vi "Go.vi"(9 "Timing Values":dbl[](array[numeric]), 10 "Control In":T1, 11 "CAD Dispense in":refnum<class "CAD Dispense.lvclass">) -> (2 "Control Out":T1, 3 "CAD Dispense Out":refnum<class "CAD Dispense.lvclass">)   [LabVIEW 2020, in "CAD Dispense.lvclass"]
uses:
  CAD Dispense.lvclass
  Controller/Motion/Motion.lvclass
  Controller/Dispenser/Dispenser.lvclass
  Aerotech.lvlib
  Program Files (x86)/Aerotech/A3200/LabVIEW/2010/Motion/MoveIncSingle.vi
  Controller/Controllers.ctl
  Controller/Controller.lvclass
  Controller/I-O/I-O.lvclass
  C:/Program Files (x86)/Aerotech/A3200/LabVIEW/2010/Bin/Aerotech.A3200.dll
  Program Files (x86)/Aerotech/A3200/LabVIEW/2010/Bin/Aerotech.A3200.dll
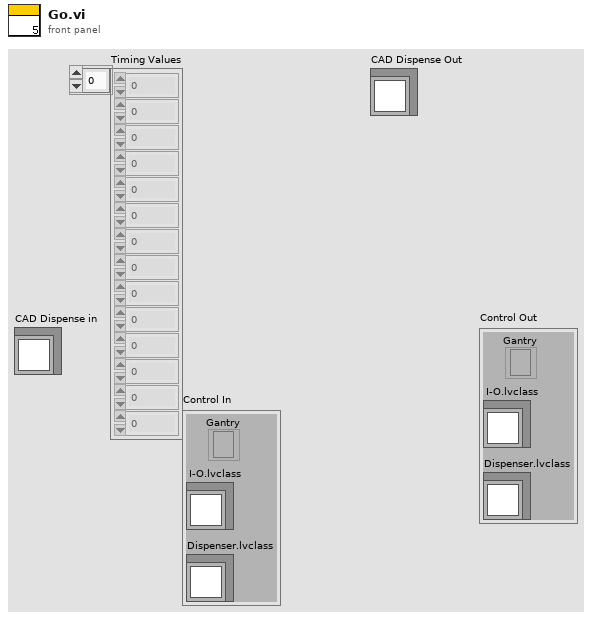
[diagram p1: front panel]
types:
  T1 = typedef "Controller.lvclass/Controllers.ctl" = cluster{"I-O.lvclass":refnum<class "I-O.lvclass">, "Dispenser.lvclass":refnum<class "Dispenser.lvclass">, "Gantry":refnum<k24>}
  T2 = cluster{"Motion":dbl[][], "Center":dbl[], "CW/CCW":dbl, "Dispense Type":enum16{"N-gon", "Square", "Arc", "Dot", "Line", "Circle"}}[]
  T3 = cluster{"Motion":dbl[][], "Center":dbl[], "CW/CCW":dbl, "Dispense Type":enum16{"N-gon", "Square", "Arc", "Dot", "Line", "Circle"}}
  T4 = typedef "ControllerDiagPacket.ctl" = cluster{"Number of Diag Packets":i32, "Axes":T5[], "error":errorcluster}
  T5 = typedef "AxisDiagPacket.ctl" = cluster{"Axis Name":string, "Analog Input 0":dbl, "Analog Input 1":dbl, "Axis Fault (num)":i32, "Axis Fault (str)":string, "Axis Fault (bits)":cluster{"AmplifierFault":bool, "AmplifierTemperatureFault":bool, "CcwEndOfTravelLimitFault":bool, "CcwSoftwareLimitFault":bool, "CommunicationLostFault":bool, "CwEndOfTravelLimitFault":bool, "CwSoftwareLimitFault":bool, "EmergencyStopFault":bool, "EncoderFault":bool, "ExternalFault":bool, "FeedbackScalingFault":bool, "GantryMisalignFault ":bool, "HallSensorFault":bool, "InPositionTimeoutFault":bool, "InternalFault":bool, "MarkerSearchFault":bool, "MaxVelocityCommandFault":bool, "MissedInterruptFault":bool, "MotorTemperatureFault":bool, "None":bool, "OverCurrentFault":bool, "PositionErrorFault":bool, "PositionFeedbackFault":bool, "PowerSupplyFault":bool, "ProbeInputFault":bool, "SafeZoneFault":bool, "VelocityErrorFault":bool, "VelocityFeedbackFault":bool, "VoltageClampFault":bool}, "Axis Status (num)":i32, "Axis Status (str)":string, "Axis Status (bits)":cluster{"BacklashActive":bool, "CalibrationEnabled1D":bool, "CalibrationEnabled2D":bool, "CommandValid":bool, "DriveAbortPending":bool, "DrivePending":bool, "Enabling":bool, "GainMappingEnabled":bool, "GantryAligned":bool, "GantryRealigning":bool, "Homed":bool, "Homing":bool, "IFOVEnabled":bool, "JogGenerating":bool, "Jogging":bool, "JoystickControl":bool, "MasterSlaveControl":bool, "MotionBlocked":bool, "MotionClamped":bool, "MoveDone":bool, "None":bool, "NotVirtual":bool, "Profiling":bool, "Stability0":bool, "Stability1":bool, "TrajectoryFiltering":bool, "WaitDone":bool}, "Current Command":sgl, "Current Error":sgl, "Current Feedback":sgl, "Digital Inputs":i32, "Digital Outputs":i32, "Drive Status":i32, "Drive Status (str)":string, "Drive Status (bits)":cluster{"AccelerationPhase":bool, "AutofocusActive":bool, "BrakeOutput":bool, "CcwEndOfTravelLimitInput":bool, "CosineEncoderError":bool, "CurrentClamp":bool, "CwEndOfTravelLimitInput":bool, "DecelerationPhase":bool, "DualLoopActive":bool, "EmergencyStopInput":bool, "Enabled":bool, "EncoderClipping":bool, "GalvoCalibrationEnabled":bool, "GalvoPowerCorrection":bool, "HallAInput":bool, "HallBInput":bool, "HallCInput":bool, "HighResolutionMode":bool, "HomeLimitInput":bool, "InPosition":bool, "InPosition2":bool, "MarkerInput":bool, "MarkerLatch":bool, "MoveActive":bool, "NoMotorSupply":bool, "None":bool, "PowerLimiting":bool, "ProgrammingFlash":bool, "ProgrammingMXH":bool, "PSOHaltLatch":bool, "ServoControl":bool, "SineEncoderError":bool}, "Position Feedback Auxiliary":dbl, "Position Command":dbl, "Position Error":dbl, "Position Feedback":dbl, "Program Position Command":dbl, "Program Position Error":dbl, "Program Position Feedback":dbl, "Velocity Command":dbl, "Velocity Error":dbl, "Velocity Feedback":dbl}
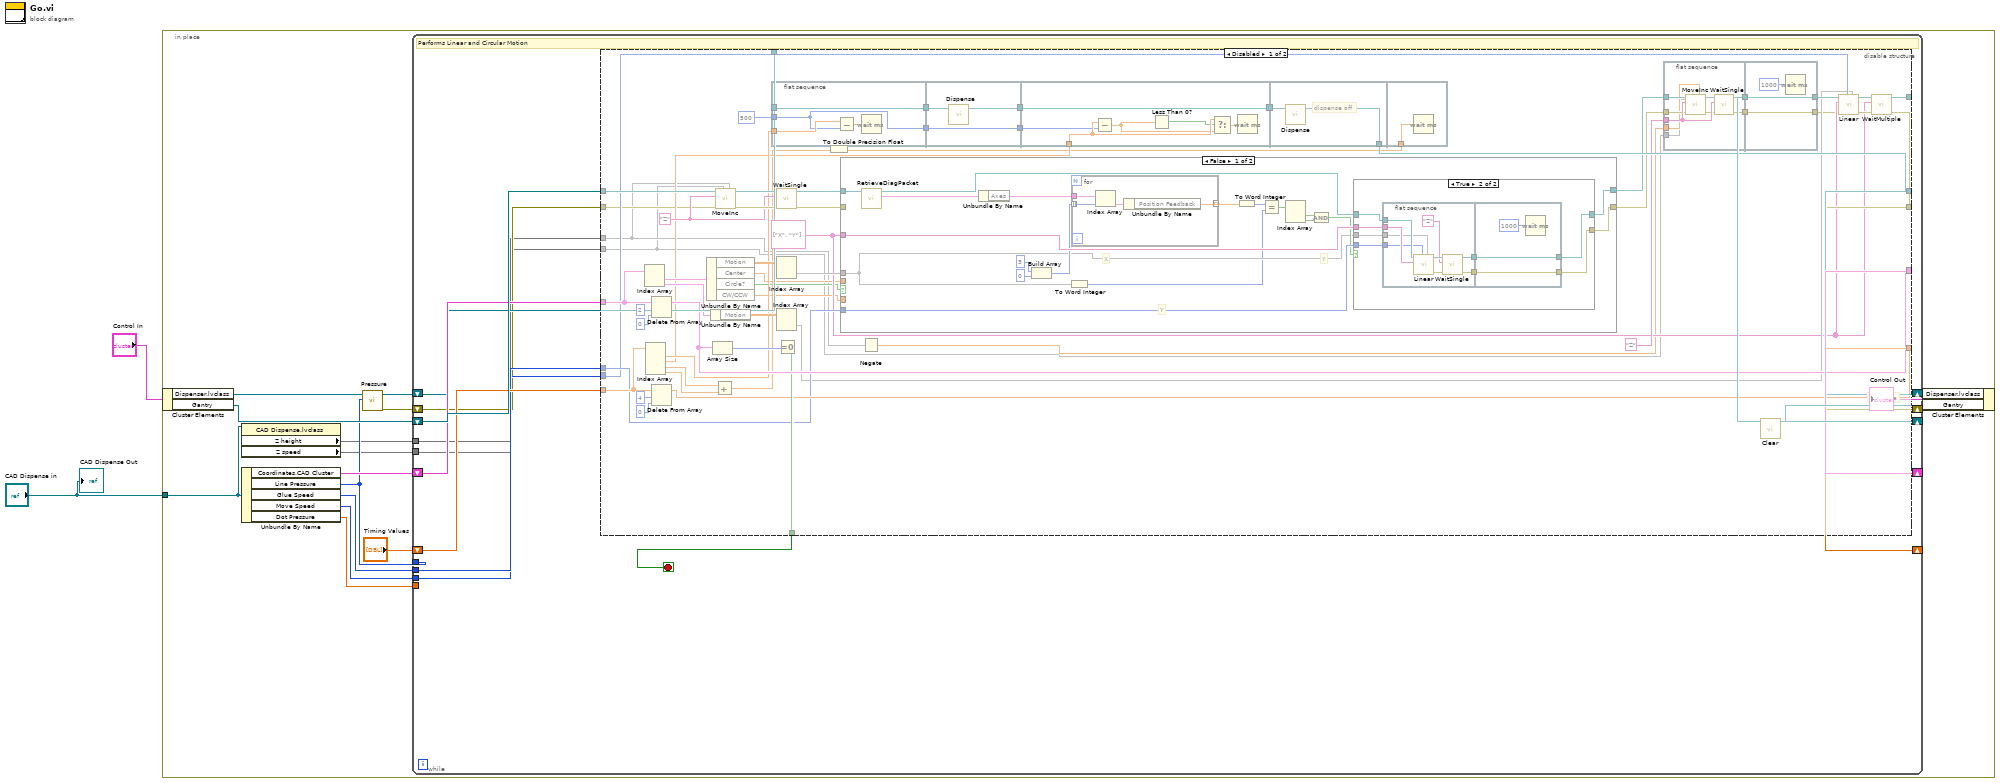
[diagram p0: block diagram]
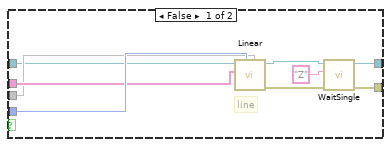
[diagram p2: hidden frame]
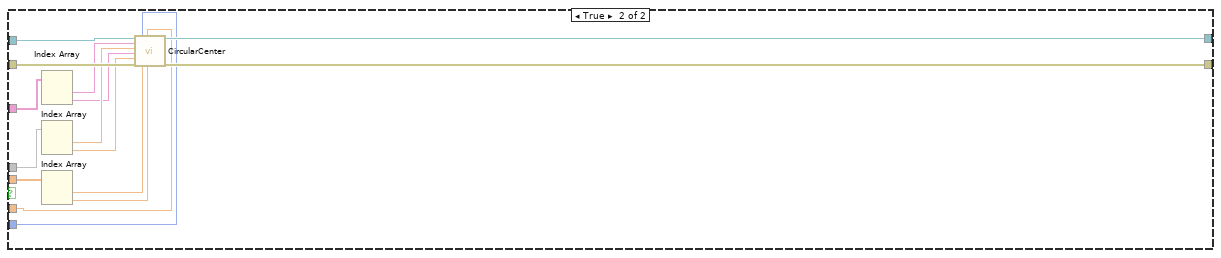
[diagram p3: hidden frame]
diagram:
  n1 = in-place {
    in-place-border: "CAD Dispense in" -> [w6]
    n2 = in-place-cluster #1("Control In") -> ("Dispenser.lvclass"=w18:refnum<class "Dispenser.lvclass">, "Gantry"=w15:refnum<k24>)
    n3 = property class="CAD Dispense.lvclass"(reference=w6) -> ("Z height"=w5, "Z speed"=w4)  [unwired: 1 in, 2 out]
    n4 = Unbundle By Name(w6) -> ("Coordinates.CAD Cluster"=w17:T2, "Line Pressure"=w7:i64, "Glue Speed"=w11:i32, "Move Speed"=w10:i32, "Dot Pressure"=w8:dbl)
    n5 = call-dynamic "Pressure.vi"("Pressure"=w7, "Dispenser in"=w18) -> ("error out"=w9:errorcluster, "Dispenser out"=w13:refnum<class "Dispenser.lvclass">)  [unwired: 8 in]
    n6 = while {
      shift-right: [w26] -> w19
      shift-left: w13 -> [w29]
      shift-right: [w30] -> w16
      shift-left: w15 -> [w34]
      shift-right: [w32] -> _
      shift-left: w17 -> [w33]
      shift-right: [w27] -> _
      shift-left: "Timing Values" -> [w28]
      tunnel: w11 -> [w25]
      tunnel: w10 -> [w24]
      shift-right: [w22] -> _
      shift-left: w9 -> [w23]
      tunnel: w8 -> [_]
      tunnel: w7 -> [_]
      tunnel: w5 -> [w21]
      tunnel: w4 -> [w20]
      stop <- w31 stop-if-true
      # "Performs Linear and Circular Motion"
      n7 = disable-structure shown="Disabled" {
        disable-tunnel: w34 -> [w83 _]
        disable-tunnel: w33 -> [w82 _]
        disable-tunnel: [w81 _] -> w32
        disable-tunnel: [w80 _] -> w31
        disable-tunnel: [w79 _] -> w30
        disable-tunnel: w29 -> [w78 _]
        disable-tunnel: w28 -> [w77 _]
        disable-tunnel: [w76 _] -> w27
        disable-tunnel: [w75 _] -> w26
        disable-tunnel: w25 -> [w74 _]
        disable-tunnel: w24 -> [w73 _]
        disable-tunnel: w23 -> [w42 _]
        disable-tunnel: [w41 _] -> w22
        disable-tunnel: w21 -> [w37 _]
        disable-tunnel: w20 -> [w35 _]
        frame Disabled {
          w55 = string[] ["X", "Y"] ("axis names")
          w61 = "Z" ("axis name")
          # "dispense"
          n8 = Index Array(array=w82) -> (element #1=w72:T3, element #2=w69:T3)  [unwired: 2 in]
          n9 = Index Array(array=w77) -> (element #1=w54:dbl, element #2=w53:dbl, element #3=w52:dbl, element #4=w51:dbl)  [unwired: 4 in]
          n10 = Delete From Array(array=w82, length=2, index=0) -> (array with subset deleted=w81:T2)  [unwired: 1 out]
          n11 = Delete From Array(array=w77, length=4, index=0) -> (array with subset deleted=w76:dbl[])  [unwired: 1 out]
          n12 = Unbundle By Name(w72) -> ("Motion"=w71:dbl[][], "Center"=w47:dbl[], "Circle?"=w46:bool, "CW/CCW"=w45:dbl)
          n13 = Unbundle By Name(w69) -> ("Motion"=w68:dbl[][])
          n14 = Array Size(array=w81) -> (size(s)=w64:i32)
          n15 = Add(x=w52, y=w51) -> (x+y=w50:dbl)
          n16 = call-poly "MoveInc.vi"("distance"=w37, "speed"=w35, "error in (no error)"=w42, "axis name"=w61, "controller in"=w83) -> ("error out"=w62:errorcluster, "controller out"=w63:refnum<k24>)  [unwired: 5 in]
          n17 = flat-sequence {
            tunnel: w54 -> [w171]
            tunnel: w78 -> [w173]
            tunnel: [w173] -> w90
            tunnel: 500 -> [w170]
            tunnel: [w170] -> w89
            tunnel: w90 -> [w176]
            tunnel: [w175] -> w88
            tunnel: w89 -> [w174]
            tunnel: [w174] -> w87
            tunnel: w53 -> [w182]
            tunnel: w88 -> [w177]
            tunnel: [w177] -> w86
            tunnel: w87 -> [w179]
            tunnel: w86 -> [w184]
            tunnel: [w183] -> w75
            tunnel: w50 -> [w185]
            frame #0 {
              n18 = Subtract(x=w171, y=w170) -> (x-y=w172:dbl)
              n19 = Wait (ms)(milliseconds to wait=w172) -> ()  [unwired: 1 out]
            }
            frame #1 {
              n20 = call-dynamic "Dispense.vi"("Dispenser in"=w176) -> ("Dispenser out"=w175:refnum<class "Dispenser.lvclass">)  [unwired: 9 in, 1 out]
            }
            frame #2 {
              n21 = Subtract(x=w182, y=w179) -> (x-y=w181:dbl)
              n22 = Less Than 0?(x=w181) -> (x < 0?=w178:bool)
              n23 = Select(t=w182, s=w178, f=w181) -> (s? t:f=w180:dbl)
              n24 = Wait (ms)(milliseconds to wait=w180) -> ()  [unwired: 1 out]
            }
            frame #3 {
              # "dispense off"
              n25 = call-dynamic "Dispense.vi"("Dispenser in"=w184) -> ("Dispenser out"=w183:refnum<class "Dispenser.lvclass">)  [unwired: 9 in, 1 out]
            }
            frame #4 {
              n26 = Wait (ms)(milliseconds to wait=w185) -> ()  [unwired: 1 out]
            }
          }
          n27 = call "WaitSingle.vi"("error in (no error)"=w62, "axis name"=w61, "controller in"=w63) -> ("error out"=w60:errorcluster, "controller out"=w38:refnum<k24>)  [unwired: 6 in, 1 out]
          n28 = Index Array(array=w71) -> (element=w70:dbl[])  [unwired: 2 in]
          n29 = Index Array(array=w68) -> (element=w67:dbl[])  [unwired: 2 in]
          n30 = Equal To 0?(x=w64) -> (x = 0?=w80:bool)
          n31 = To Double Precision Float() -> ()  [unwired: 1 in, 1 out]
          n32 = case shown="False" w46 {
            tunnel: w74 -> [w121 w165]
            tunnel: w70 -> [w106 w160]
            tunnel: w60 -> [_ w168]
            tunnel: [w118 w169] -> w40
            tunnel: [w120 w167] -> w39
            tunnel: w55 -> [w119 w166]
            tunnel: w47 -> [_ w163]
            tunnel: w45 -> [_ w164]
            tunnel: w38 -> [w107 w155]
            frame False {
              # "Y"
              # "X"
              # "Y"
              n33 = call "RetrieveDiagPacket.vi"("Controller In"=w107) -> ("ControllerDiagPacket"=w117:T4, "Controller Out"=w108:refnum<k24>)  [unwired: 8 in, 1 out]
              n34 = Unbundle By Name(w117) -> ("Axes"=w116:T5[])
              n35 = Build Array(3, 0) -> (w115:i32[])
              n36 = To Word Integer(number=w106) -> (16bit integer=w103:i16[])
              n37 = for {
                tunnel: w116 -> [w124]
                tunnel: [w125] -> w105 mode=indexing
                tunnel: w115 -> [w122] mode=indexing
                n38 = Index Array(array=w124, index=w122) -> (element=w123:T5)
                n39 = Unbundle By Name(w123) -> ("Position Feedback"=w125:dbl)
              }
              n40 = To Word Integer(number=w105) -> (16bit integer=w104:i16[])
              n41 = Equal?(x=w104, y=w103) -> (x = y?=w112:bool[])
              n42 = Index Array(array=w112) -> (element #1=w111:bool, element #2=w110:bool)  [unwired: 2 in]
              n43 = And(x=w111, y=w110) -> (x .and. y?=w109:bool)
              n44 = case shown="True" w109 {
                tunnel: w121 -> [w134 w139]
                tunnel: [w133 w135] -> w120
                tunnel: w119 -> [w132 w141]
                tunnel: [w131 w137] -> w118
                tunnel: w106 -> [w130 w140]
                tunnel: w108 -> [w126 w142]
                frame False {
                  # "line"
                  n45 = call "Linear.vi"("distances"=w130, "speed"=w134, "axis names"=w132, "controller in"=w126) -> ("error out"=w127:errorcluster, "controller out"=w129:refnum<k24>)  [unwired: 6 in]
                  n46 = call "WaitSingle.vi"("error in (no error)"=w127, "axis name"="Z", "controller in"=w129) -> ("error out"=w133:errorcluster, "controller out"=w131:refnum<k24>)  [unwired: 6 in, 1 out]
                }
                frame True {
                  n47 = flat-sequence {
                    tunnel: w142 -> [w148]
                    tunnel: w141 -> [w147]
                    tunnel: w140 -> [w146]
                    tunnel: w139 -> [w145]
                    tunnel: [w144] -> w138
                    tunnel: [w143] -> w136
                    tunnel: w138 -> [w153]
                    tunnel: [w153] -> w137
                    tunnel: w136 -> [w152]
                    tunnel: [w152] -> w135
                    frame #0 {
                      n48 = call "Linear.vi"("distances"=w146, "speed"=w145, "axis names"=w147, "controller in"=w148) -> ("error out"=w149:errorcluster, "controller out"=w151:refnum<k24>)  [unwired: 6 in]
                      n49 = call "WaitSingle.vi"("error in (no error)"=w149, "axis name"="Z", "controller in"=w151) -> ("error out"=w143:errorcluster, "controller out"=w144:refnum<k24>)  [unwired: 6 in, 1 out]
                    }
                    frame #1 {
                      n50 = Wait (ms)(milliseconds to wait=u32 1000) -> ()  [unwired: 1 out]
                    }
                  }
                }
              }
            }
            frame True {
              n51 = Index Array(array=w166) -> (element #1=w157:string, element #2=w156:string)  [unwired: 2 in]
              n52 = Index Array(array=w160) -> (element #1=w159:dbl, element #2=w158:dbl)  [unwired: 2 in]
              n53 = Index Array(array=w163) -> (element #1=w162:dbl, element #2=w161:dbl)  [unwired: 2 in]
              n54 = call "CircularCenter.vi"("controller in"=w155, "axis 1 name"=w157, "axis 1 endpoint"=w159, "axis 2 name"=w156, "axis 2 endpoint"=w158, "error in (no error)"=w168, "speed"=w165, "axis 1 center point"=w162, "direction"=w164, "axis 2 center point"=w161) -> ("controller out"=w169:refnum<k24>, "error out"=w167:errorcluster)  [unwired: 8 in]
            }
          }
          n55 = Negate(x=w37) -> (-x=w36:dbl)
          n56 = flat-sequence {
            tunnel: "Z" ("axis name") -> [w97]
            tunnel: w40 -> [w94]
            tunnel: w39 -> [w93]
            tunnel: [w98] -> w85
            tunnel: [w95] -> w84
            tunnel: w36 -> [w92]
            tunnel: w35 -> [w91]
            tunnel: [w101] -> w43
            tunnel: [w102] -> w59
            tunnel: w85 -> [w102]
            tunnel: w84 -> [w101]
            frame #0 {
              n57 = call-poly "MoveInc.vi"("distance"=w92, "speed"=w91, "error in (no error)"=w93, "axis name"=w97, "controller in"=w94) -> ("error out"=w96:errorcluster, "controller out"=w99:refnum<k24>)  [unwired: 5 in]
              n58 = call "WaitSingle.vi"("error in (no error)"=w96, "axis name"=w97, "controller in"=w99) -> ("error out"=w95:errorcluster, "controller out"=w98:refnum<k24>)  [unwired: 6 in, 1 out]
            }
            frame #1 {
              n59 = Wait (ms)(milliseconds to wait=1000) -> ()  [unwired: 1 out]
            }
          }
          n60 = call "Linear.vi"("distances"=w67, "speed"=w73, "error in (no error)"=w43, "axis names"=w55, "controller in"=w59) -> ("error out"=w57:errorcluster, "controller out"=w56:refnum<k24>)  [unwired: 5 in]
          n61 = call "WaitMultiple.vi"("error in (no error)"=w57, "axis names"=w55, "controller in"=w56) -> ("error out"=w41:errorcluster, "controller out"=w79:refnum<k24>)  [unwired: 6 in, 1 out]
        }
        frame Enabled {
          n62 = flat-sequence {
            frame #0 {
            }
          }
        }
      }
    }
    n63 = call "Clear.vi"("Gantry 2"=w16) -> ("Gantry 3"=w14:refnum<k24>)  [unwired: 9 in, 1 out]
    n64 = in-place-cluster #1("Dispenser.lvclass"=w19, "Gantry"=w14) -> (→"Control Out":T1)
  }
  "CAD Dispense Out" <- "CAD Dispense in"
